vi "多参数数据插入.vi"(8 "error in (no error)":errorcluster caption="错误输入（无错误）", 9 "编号":string, 10 "columns enable":T1, 11 "data in":T2) -> (0 "error out":errorcluster)   [LabVIEW 2016, in "斯坦道多参数.lvlib"]
uses:
  <vilib>/addons/database/Auxilliary.llb/DB Tools Column Info.ctl
  <vilib>/addons/database/Auxilliary.llb/DB Tools DataTypes.ctl
  <vilib>/addons/database/NI_Database_API.lvlib
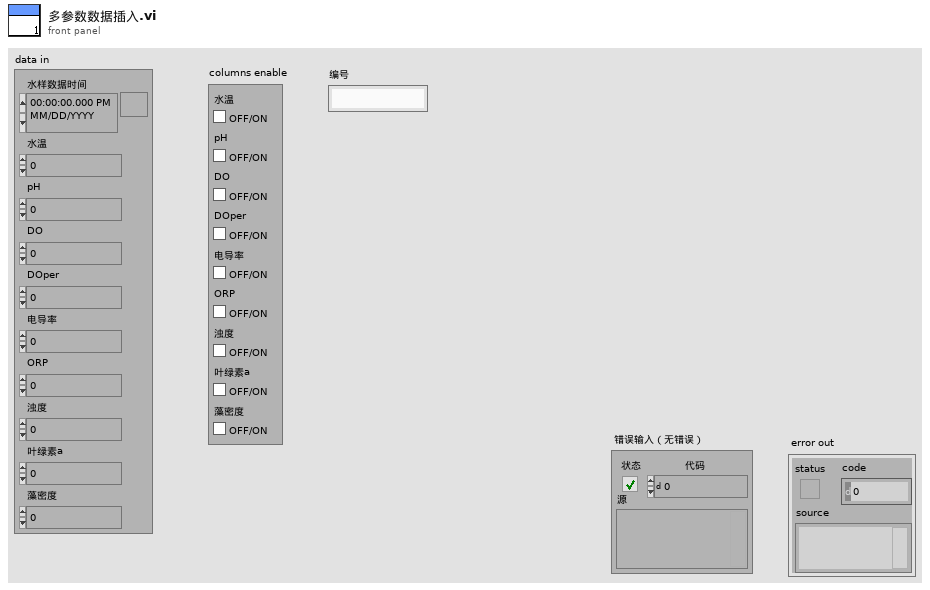
[diagram p1: front panel]
types:
  T1 = cluster{"水温":bool, "pH":bool, "DO":bool, "DOper":bool, "电导率":bool, "ORP":bool, "浊度":bool, "叶绿素a":bool, "藻密度":bool}
  T2 = cluster{"水样数据时间":timestamp, "水温":dbl, "pH":dbl, "DO":dbl, "DOper":dbl, "电导率":dbl, "ORP":dbl, "浊度":dbl, "叶绿素a":dbl, "藻密度":dbl}
  T3 = typedef "NI_Database_API.lvlib/DB Tools Column Info.ctl" = cluster{"column name":string, "data type":T4, "size":i32, "allow null?":bool}
  T4 = typedef "NI_Database_API.lvlib/DB Tools DataTypes.ctl" = enum16{"String", "Long (I32)", "Single (SGL)", "Double (DBL)", "Date/Time", "Binary"}
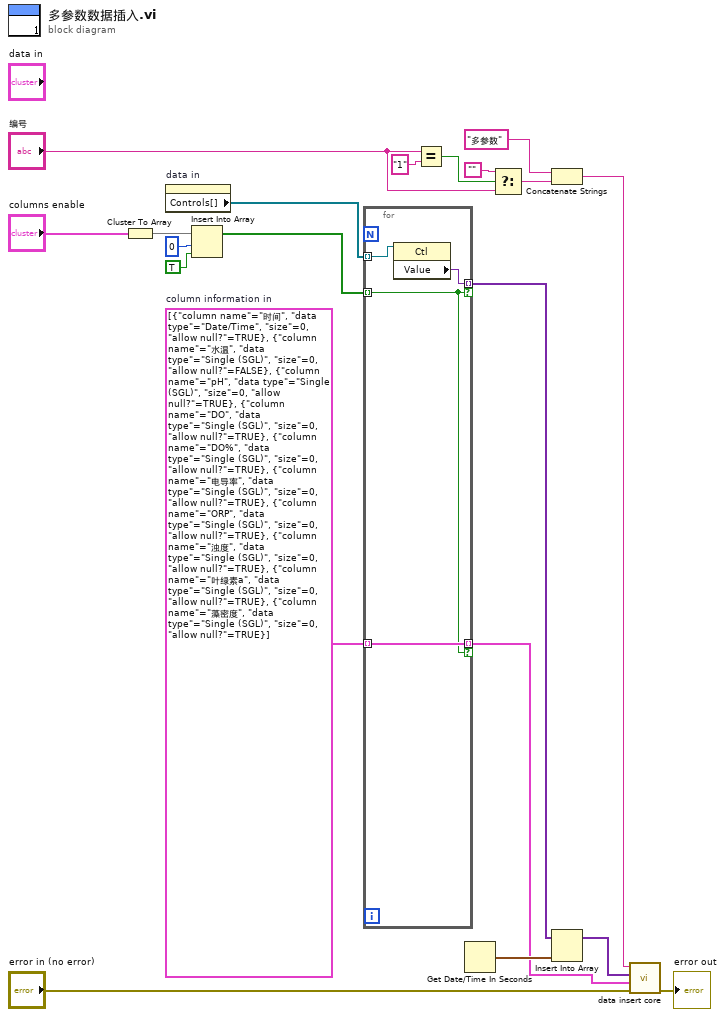
[diagram p0: block diagram]
diagram:
  w8 = T3[] [{"column name"="时间", "data type"=enum."Date/Time", "size"=0, "allow null?"=TRUE}, {"column name"="水温", "data type"=enum."Single (SGL)", "size"=0, "allow null?"=FALSE}, {"column name"="pH", "data type"=enum."Single (SGL)", "size"=0, "allow null?"=TRUE}, {"column name"="DO", "data type"=enum."Single (SGL)", "size"=0, "allow null?"=TRUE}, {"column name"="DO%", "data type"=enum."Single (SGL)", "size"=0, "allow null?"=TRUE}, {"column name"="电导率", "data type"=enum."Single (SGL)", "size"=0, "allow null?"=TRUE}, {"column name"="ORP", "data type"=enum."Single (SGL)", "size"=0, "allow null?"=TRUE}, {"column name"="浊度", "data type"=enum."Single (SGL)", "size"=0, "allow null?"=TRUE}, {"column name"="叶绿素a", "data type"=enum."Single (SGL)", "size"=0, "allow null?"=TRUE}, {"column name"="藻密度", "data type"=enum."Single (SGL)", "size"=0, "allow null?"=TRUE}]  # column information in
  n1 = Cluster To Array(cluster="columns enable") -> (array=w3:bool[])
  n2 = property on="data in" class="Clust (严格)"() -> ("Controls[]"=w12:refnum<vi>[])  [unwired: 2 in, 2 out]
  n3 = Insert Into Array(array=w3, index=0 ("索引"), new element=TRUE ("新元素/子数组")) -> (w4:bool[])
  n4 = for {
    tunnel: w12 -> [w24] mode=indexing
    tunnel: [w23] -> w11 mode=indexing if=w21
    tunnel: w8 -> [w22] mode=indexing
    tunnel: [w22] -> w7 mode=indexing if=w21
    tunnel: w4 -> [w21] mode=indexing
    n5 = property class="Ctl"(reference=w24) -> ("Value"=w23:variant)  [unwired: 1 in, 2 out]
  }
  n6 = Equal?(x="编号", y="1") -> (x = y?=w17:bool)
  n7 = Get Date/Time In Seconds() -> (seconds since 1Jan1904=w10:timestamp)
  n8 = Select(t="", s=w17, f="编号") -> (s? t:f=w14:string)
  n9 = Concatenate Strings("多参数" ("字符串"), w14) -> (w13:string)
  n10 = Insert Into Array(array=w11, new element=w10) -> (w9:variant[])  [unwired: 1 in]
  n11 = call "data insert core.vi"("error in (no error)"="error in (no error)", "column information"=w7, "data"=w9, "table"=w13) -> ("error out"=→"error out":errorcluster)  [unwired: 7 in]
